vi "8-ModifyNIAFClass.vi"   [LabVIEW 2016, in "TestVIs.lvlib"]
uses:
  TestVIs.lvlib
types:
  T1 = enum16{"Invalid Wire Rule", "Required", "Recommended", "Optional", "Dynamic Dispatch"}
  T2 = typedef "LVRectTypeDef.ctl" = cluster{"Left":i16, "Top":i16, "Right":i16, "Bottom":i16}
  T3 = enum16{"Invalid Wire Rule", "Required", "Recommended", "Optional", "Dynamic Dispatch"}[]
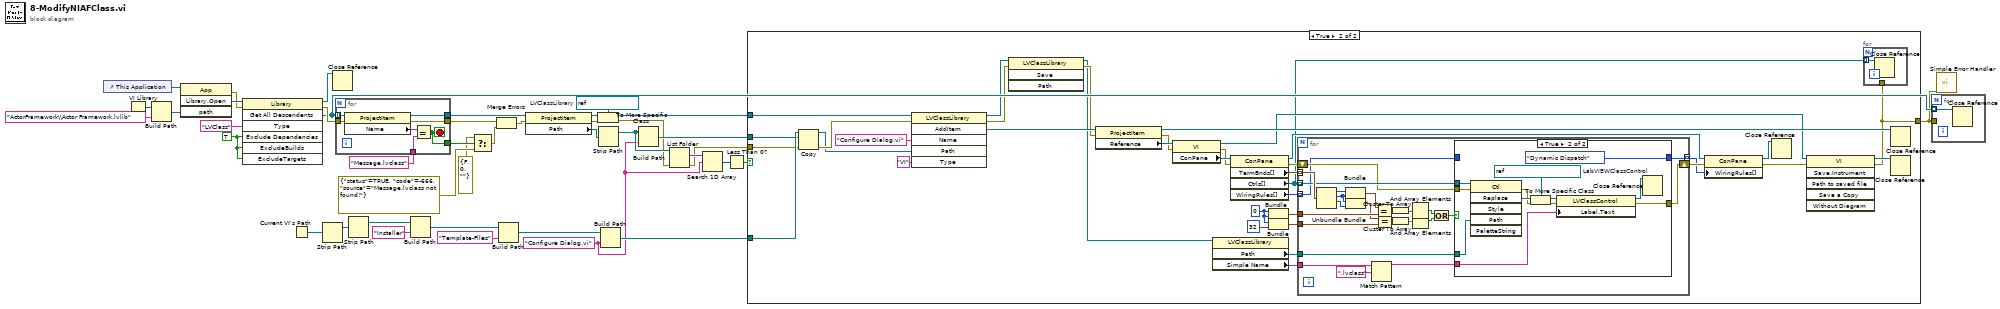
[diagram p0: block diagram]
diagram:
  w15 = refnum<vi> refnum  # LVClassLibrary
  w4 = "Configure Dialog.vi" ("name or relative path")
  w34 = TRUE ("ExcludeDependencies")
  n1 = control-ref of="This Application"() -> (w41:refnum<vi>)
  n2 = VI Library() -> (path=w40:path)
  n3 = Build Path(base path=w40, name or relative path="ActorFramework\\Actor Framework.lvlib") -> (appended path=w38:path)
  n4 = invoke class="App" method="Library.Open"(reference=w41, "path"=w38) -> (error out=w35:errorcluster, "Open Library"=w36:refnum<vi>)  [unwired: 2 in, 2 out]
  n5 = invoke class="Library" method="Get All Descendents"(reference=w36, error in=w35, "Type"="LVClass", "Exclude Dependencies"=w34, "ExcludeBuilds"=w34, "ExcludeTargets"=w34) -> (reference out=w11:refnum<vi>, error out=w33:errorcluster, "All Descendents"=w10:refnum<vi>[])  [unwired: 1 in, 4 out]
  n6 = Current VI's Path() -> (path=w26:path)
  n7 = Strip Path(path=w26) -> (stripped path=w25:path)  [unwired: 1 out]
  n8 = Close Reference(reference=w11) -> ()  [unwired: 1 in, 1 out]
  n9 = for {
    tunnel: w10 -> [w48] mode=indexing
    tunnel: "Message.lvclass" ("name") -> [w46]
    tunnel: [w45] -> w19
    tunnel: w33 -> [w44]
    tunnel: [w43] -> w27
    tunnel: [w42] -> w31
    stop <- w42 stop-if-true
    n10 = property class="ProjectItem"(reference=w48, error in=w44) -> (reference out=w45:refnum<vi>, error out=w43:errorcluster, "Name"=w47:string)
    n11 = Equal?(x=w47, y=w46) -> (x = y?=w42:bool)
  }
  n12 = Strip Path(path=w25) -> (stripped path=w24:path)  [unwired: 1 out]
  n13 = Build Path(base path=w24, name or relative path="Installer") -> (appended path=w21:path)
  n14 = Select(t=errorcluster {"status"=FALSE, "code"=0, "source"=""} ("error constant"), s=w31, f=errorcluster {"status"=TRUE, "code"=-666, "source"="Message.lvclass not found!"} ("error constant")) -> (s? t:f=w28:errorcluster)
  n15 = Merge Errors(w27, w28) -> (w18:errorcluster)
  n16 = Build Path(base path=w21, name or relative path="Template-Files") -> (appended path=w20:path)
  n17 = property class="ProjectItem"(reference=w19, error in=w18) -> (reference out=w14:refnum<vi>, error out=w12:errorcluster, "Path"=w16:path)
  n18 = To More Specific Class(target class=w15, reference=w14, error in=w12) -> (specific class reference=w13:refnum<vi>, error out=w6:errorcluster)
  n19 = Strip Path(path=w16) -> (stripped path=w7:path)  [unwired: 1 out]
  n20 = Build Path(base path=w20, name or relative path=w4) -> (appended path=w17:path)
  n21 = Build Path(base path=w7, name or relative path=w4) -> (appended path=w8:path)
  n22 = List Folder(path=w7, error in=w6) -> (filenames=w5:string[], error out=w3:errorcluster)  [unwired: 2 in, 2 out]
  n23 = Search 1D Array(1D array=w5, element=w4) -> (index of element=w2:i32)  [unwired: 1 in]
  n24 = Less Than 0?(x=w2) -> (x < 0?=w1:bool)
  n25 = case shown="True" w1 {
    tunnel: w17 -> [_ w79]
    tunnel: w13 -> [_ w77]
    tunnel: [w49 w52] -> w9
    tunnel: w8 -> [_ w51]
    tunnel: w3 -> [w49 w50]
    frame False {
    }
    frame True {
      w65 = i16 0
      n26 = Copy(8:w50, 10:w51, 11:w79) -> (0:w80:errorcluster, 3:w78:path)  [unwired: 2 in, 1 out]
      n27 = invoke class="LVClassLibrary" method="AddItem"(reference=w77, error in=w80, "Name"="Configure Dialog.vi", "Path"=w78, "Type"="VI") -> (reference out=w76:refnum<vi>, error out=w75:errorcluster, "AddItem"=w83:refnum<vi>)  [unwired: 1 in, 3 out]
      n28 = invoke class="LVClassLibrary" method="Save"(reference=w76, error in=w75) -> (reference out=w57:refnum<vi>, error out=w74:errorcluster)  [unwired: 2 in, 2 out]
      n29 = property class="ProjectItem"(reference=w83, error in=w74) -> (reference out=w82:refnum<vi>, error out=w58:errorcluster, "Reference"=w59:refnum<vi>)
      n30 = property class="VI"(reference=w59, error in=w58) -> (reference out=w56:refnum<vi>, error out=w72:errorcluster, "ConPane"=w73:refnum<vi>)
      n31 = property class="LVClassLibrary"(reference=w57) -> ("Path"=w66:path, "Simple Name"=w60:string)  [unwired: 1 in, 2 out]
      n32 = property class="ConPane"(reference=w73, error in=w72) -> (reference out=w62:refnum<vi>, error out=w70:errorcluster, "TermBnds[]"=w71:T2[], "Ctrls[]"=w53:refnum<vi>[], "WiringRules[]"=w64:T3)
      n33 = Bundle(w65, w65) -> (w68:cluster{i16, i16})  [unwired: 1 in]
      n34 = Bundle(w65, i16 32) -> (w67:cluster{i16, i16})  [unwired: 1 in]
      n35 = for {
        tunnel: w71 -> [w109] mode=indexing
        tunnel: w53 -> [w99] mode=indexing
        shift-right: [w93] -> w63
        shift-left: w70 -> [w98]
        tunnel: w68 -> [w106]
        tunnel: w67 -> [w104]
        tunnel: w66 -> [w94]
        tunnel: w64 -> [w90] mode=indexing
        tunnel: [w89] -> w61 mode=indexing
        tunnel: w60 -> [w88]
        n36 = Unbundle(w109) -> ("Left"=w108:i16, "Top"=w91:i16, "Right"=w92:i16)  [unwired: 1 out]
        n37 = Bundle("Left"=w108, "Top"=w91) -> (w107:cluster{"Left":i16, "Top":i16})  [unwired: 1 in]
        n38 = Bundle("Top"=w91, "Right"=w92) -> (w105:cluster{"Top":i16, "Right":i16})  [unwired: 1 in]
        n39 = Match Pattern(string=w88, regular expression=".lvclass") -> (before substring=w87:string)  [unwired: 1 in, 3 out]
        n40 = Equal?(x=w107, y=w106) -> (x = y?=w103:cluster{bool, bool})
        n41 = Equal?(x=w105, y=w104) -> (x = y?=w102:cluster{bool, bool})
        n42 = Cluster To Array(cluster=w103) -> (array=w101:bool[])
        n43 = Cluster To Array(cluster=w102) -> (array=w100:bool[])
        n44 = And Array Elements(Boolean array=w101) -> (logical AND=w97:bool)
        n45 = And Array Elements(Boolean array=w100) -> (logical AND=w96:bool)
        n46 = Or(x=w97, y=w96) -> (x .or. y?=w95:bool)
        n47 = case shown="True" w95 {
          tunnel: w99 -> [_ w123]
          tunnel: w98 -> [w111 w122]
          tunnel: [w111 w114] -> w93
          tunnel: w94 -> [_ w121]
          tunnel: w90 -> [w110 _]
          tunnel: [w110 T1."Dynamic Dispatch" ("Wire Rule")] -> w89
          tunnel: w87 -> [_ w112]
          frame False {
          }
          frame True {
            w119 = refnum<vi> refnum  # LabVIEWClassControl
            n48 = invoke class="Ctl" method="Replace"(reference=w123, error in=w122, "Path"=w121) -> (error out=w115:errorcluster, "Replace"=w118:refnum<vi>)  [unwired: 3 in, 4 out]
            n49 = To More Specific Class(target class=w119, reference=w118, error in=w115) -> (specific class reference=w117:refnum<vi>, error out=w116:errorcluster)
            n50 = property class="LVClassControl"(reference=w117, error in=w116, "Label.Text"=w112) -> (reference out=w113:refnum<vi>, error out=w114:errorcluster)
            n51 = Close Reference(reference=w113) -> ()  [unwired: 1 in, 1 out]
          }
        }
      }
      n52 = property class="ConPane"(reference=w62, error in=w63, "WiringRules[]"=w61) -> (reference out=w54:refnum<vi>, error out=w55:errorcluster)
      n53 = Close Reference(reference=w54) -> ()  [unwired: 1 in, 1 out]
      n54 = invoke class="VI" method="Save.Instrument"(reference=w56, error in=w55) -> (reference out=w81:refnum<vi>, error out=w52:errorcluster)  [unwired: 4 in, 4 out]
      n55 = for {
        tunnel: w53 -> [w124] mode=indexing
        tunnel: w52 -> [_]
        n56 = Close Reference(reference=w124) -> ()  [unwired: 1 in, 1 out]
      }
      n57 = Close Reference(reference=w82) -> ()  [unwired: 1 in, 1 out]
      n58 = Close Reference(reference=w81) -> ()  [unwired: 1 in, 1 out]
    }
  }
  n59 = for {
    tunnel: w9 -> [_]
    tunnel: w10 -> [w125] mode=indexing
    n60 = Close Reference(reference=w125) -> ()  [unwired: 1 in, 1 out]
  }
  n61 = call <vilib>:"Simple Error Handler.vi"("error in (no error)"=w9) -> ()  [unwired: 4 in, 5 out]
